vi "CTRE_PigeonIMU_SetStatusFrameRate.vi"(6 "timeoutMs":u32, 8 "error in (no error)":errorcluster, 9 "StatusFrame":T1=2 items=["CondStatus_1_General"=2, "CondStatus_9_SixDeg_YPR"=3, "CondStatus_6_SensorFusion"=4, "CondStatus_11_GyroAccum"=5, "CondStatus_2_GeneralCompass"=11, "CondStatus_3_GeneralAccel"=12, "CondStatus_10_SixDeg_Quat"=14, "RawStatus_4_Mag"=6, "BiasedStatus_2_Gyro"=8, "BiasedStatus_4_Mag"=9, "BiasedStatus_6_Accel"=10], 10 "Period (ms)":i16, 11 "PigeonIMUDevRef":T2={"DeviceStatus"={"status"=FALSE, "code"=0, "source"=""}, "Device Number"=0, "Type"=352321536, "Device ID"=0, "Handle"=0, "UsageFrame"=0, "Library Path"=path ""} {"Type" items=["CAN"=352321536, "TalonSRX"=33554432]}) -> (0 "error out":errorcluster, 3 "PigeonIMUDevRef":T2={"DeviceStatus"={"status"=FALSE, "code"=0, "source"=""}, "Device Number"=0, "Type"=352321536, "Device ID"=0, "Handle"=0, "UsageFrame"=0, "Library Path"=path ""} {"Type" items=["CAN"=352321536, "TalonSRX"=33554432]})   [LabVIEW 2017]
doc: "Period (ms) sets the rate at which StatusFrame is sent."
uses:
  CTRE_PigeonIMU_DeviceRef.ctl
  CTRE_PigeonIMU_ConnectionType.ctl
  CTRE_PigeonIMU_StatusFrameRate.ctl
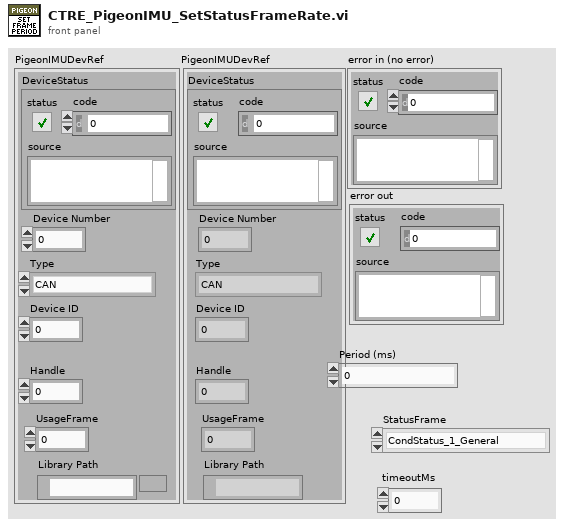
[diagram p1: front panel]
types:
  T1 = typedef "CTRE_PigeonIMU_StatusFrameRate.ctl" = u16
  T2 = typedef "CTRE_PigeonIMU_DeviceRef.ctl" = cluster{"DeviceStatus":errorcluster, "Device Number":u8, "Type":T3, "Device ID":u32, "Handle":u64, "UsageFrame":u32, "Library Path":path}
  T3 = typedef "CTRE_PigeonIMU_ConnectionType.ctl" = u32
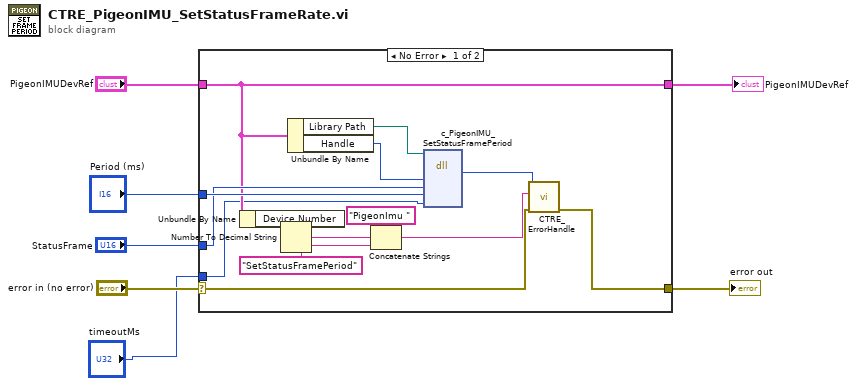
[diagram p0: block diagram]
diagram:
  n1 = case shown="No Error" "error in (no error)" {
    selector: "error in (no error)" -> [w10 w22]
    tunnel: [w9 w22] -> w6
    tunnel: [w12 w23] -> w4
    tunnel: "PigeonIMUDevRef" -> [w12 w23]
    tunnel: "Period (ms)" -> [w19 _]
    tunnel: "StatusFrame" -> [w18 _]
    tunnel: "timeoutMs" -> [w8 _]
    frame No Error {
      n2 = Unbundle By Name(w12) -> ("Device Number"=w16:u8)
      n3 = Number To Decimal String(number=w16) -> (decimal integer string=w15:string)  [unwired: 1 in]
      n4 = Unbundle By Name(w12) -> ("Library Path"=w21:path, "Handle"=w20:u64)
      n5 = Concatenate Strings("PigeonImu " ("string"), w15, "SetStatusFramePeriod" ("string")) -> (w11:string)
      n6 = dll-call lib="?" fn="c_PigeonIMU_SetStatusFramePeriod"(path in=w21, "handle"=w20, "statusFrame"=w18, "periodMs"=w19, "timeoutms"=w8) -> ("return type"=w17:i32)  [unwired: 6 in, 2 out]
      n7 = call "CTRE_ErrorHandle.vi"("error in"=w10, "origin"=w11, "code"=w17) -> ("error out"=w9:errorcluster)  [unwired: 8 in]
    }
    frame Error {
    }
  }
  "PigeonIMUDevRef" <- w4
  "error out" <- w6
